vi "TESTShell_for Inst_IO.vi"() -> ()   [LabVIEW 2010]
uses:
  <vilib>/Utility/config.llb/NI_LVConfig.lvlib
panel:
  in  "configuration file path":path
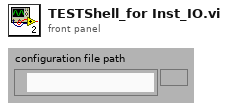
[diagram p1: front panel]
types:
  T1 = typedef "NI_LVConfig.lvlib/Config Data RefNum.ctl" = refnum<k1>
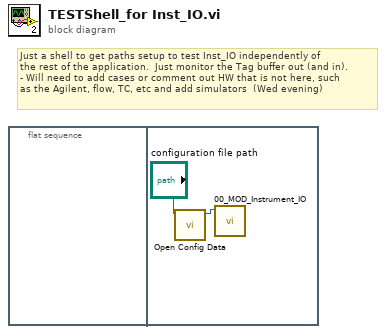
[diagram p0: block diagram]
diagram:
  # "Just a shell to get paths setup to test Inst_IO independently of\nthe rest of the application.  Just monitor the Tag buffer out (and in).\n- Will need to add cases or comment out HW that is not here, such\nas the Agilent, flow, TC, etc and add simulators  (Wed evening)"
  n1 = flat-sequence {
    frame #0 {
    }
    frame #1 {
      n2 = call <vilib>:"Open Config Data.vi"("configuration file path"="configuration file path") -> ("refnum"=w1:T1)  [unwired: 8 in, 2 out]
      n3 = call "00_MOD_Instrument_IO.vi"("Main Config File Refnum"=w1) -> ()  [unwired: 10 in, 1 out]
    }
  }
